vi "DiscriminantAnalysis.vi"   [LabVIEW 2020]
doc: "Polymorphic VI for discriminant analysis"
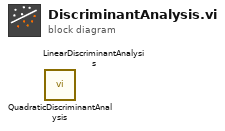
[diagram p0: block diagram]
diagram:
  n1 = call "QuadraticDiscriminantAnalysis.vi"() -> ()  [unwired: 10 in, 2 out]
  n2 = call "LinearDiscriminantAnalysis.vi"() -> ()  [unwired: 10 in, 2 out]
